vi "Timer Pause.vi"(8 "error in (no error)":errorcluster, 11 "LV Server in":refnum<class "LV Server.lvclass">) -> (0 "error out":errorcluster, 3 "LV Server out":refnum<class "LV Server.lvclass">)   [LabVIEW 2020, in "LV Server.lvclass"]
uses:
  LV Server.lvclass
  LV Server.lvclass/LV Server.ctl
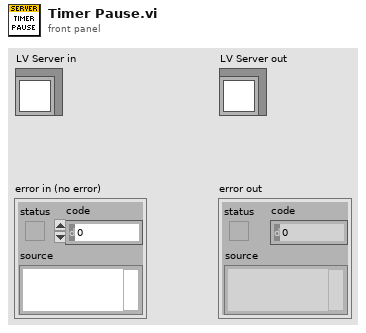
[diagram p1: front panel]
types:
  T1 = typedef "LV Server.lvclass/Timer Data.ctl" = cluster{"Start":dbl, "Accumulated":dbl, "Running":bool}
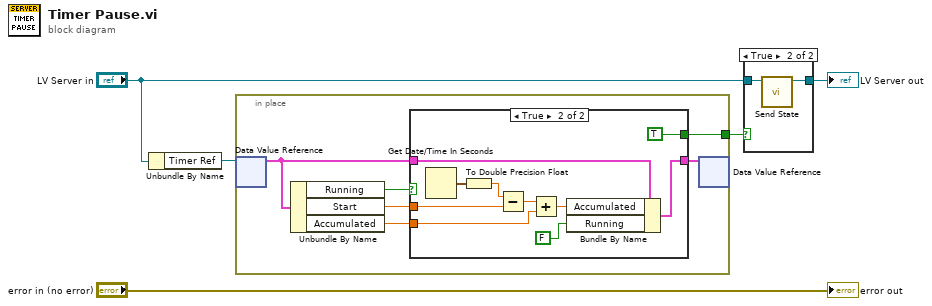
[diagram p0: block diagram]
diagram:
  n1 = Unbundle By Name("LV Server in") -> ("Timer Ref"=w4:refnum<data-value>)
  n2 = in-place {
    in-place-border: [w6] -> w2
    n3 = in-place-dvr #1(w4) -> (w10:T1)  [unwired: 1 out]
    n4 = Unbundle By Name(w10) -> ("Running"=w9:bool, "Start"=w8:dbl, "Accumulated"=w7:dbl)
    n5 = case shown="True" w9 {
      tunnel: [w12 w22] -> w11
      tunnel: w10 -> [w12 w19]
      tunnel: w8 -> [_ w18]
      tunnel: w7 -> [_ w15]
      tunnel: [_ TRUE] -> w6
      frame False {
      }
      frame True {
        n6 = Get Date/Time In Seconds() -> (seconds since 1Jan1904=w20:timestamp)
        n7 = To Double Precision Float(number=w20) -> (double precision float=w17:dbl)
        n8 = Subtract(x=w17, y=w18) -> (x-y=w16:dbl)
        n9 = Add(x=w16, y=w15) -> (x+y=w14:dbl)
        n10 = Bundle By Name(cluster=w19, "Accumulated"=w14, "Running"=FALSE) -> (w22:T1)
      }
    }
    n11 = in-place-dvr #1(w11) -> ()  [unwired: 2 out]
  }
  n12 = case shown="True" w2 {
    tunnel: "LV Server in" -> [w23 w25]
    tunnel: [w23 w24] -> w3
    frame False {
    }
    frame True {
      n13 = call "Send State.vi"("LV Server in"=w25) -> ("LV Server out"=w24:refnum<class "LV Server.lvclass">)  [unwired: 9 in, 1 out]
    }
  }
  "LV Server out" <- w3
  "error out" <- "error in (no error)"
